vi "Get RelativePath.vi"(8 "error in (no error)":errorcluster caption="错误输入（无错误）", 11 "PanelRootNode 输入":refnum<class "PanelRootNode.lvclass"> caption="DNL_LabVIEW Object in") -> (0 "error out":errorcluster caption="错误输出", 2 "RelativePath":string, 3 "PanelRootNode 输出":refnum<class "PanelRootNode.lvclass"> caption="DNL_LabVIEW Object out")   [LabVIEW 2016, in "PanelRootNode.lvclass"]
uses:
  PanelRootNode.lvclass
  C:/Users/CL/Desktop/ZcDAQprj0811/ZcDAQprj/Modules/DAQ-Display/PanelSplitToolkit/PanelDataNode/PanelDataNode.lvclass
  PanelDataNode/PanelDataNode.lvclass/PanelDataNode.ctl
  PanelDataNode/PanelDataNode.lvclass
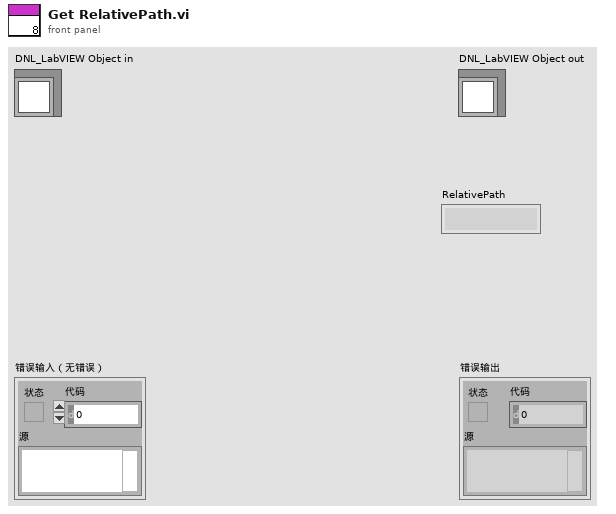
[diagram p1: front panel]
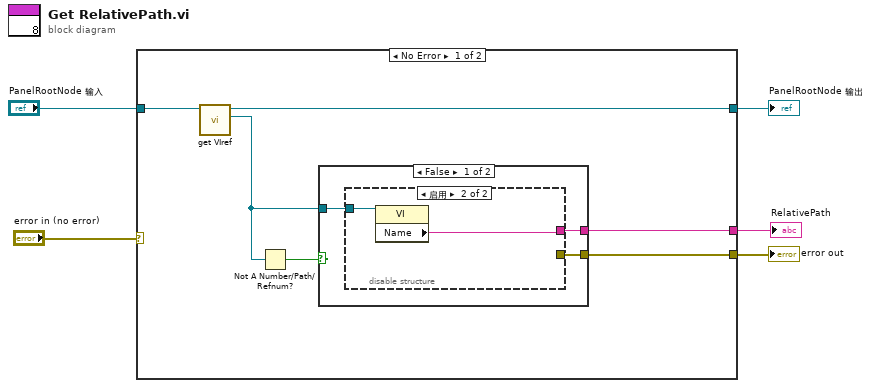
[diagram p0: block diagram]
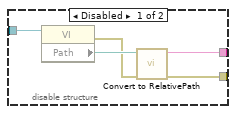
[diagram p2: hidden frame]
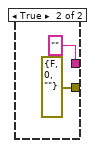
[diagram p3: hidden frame]
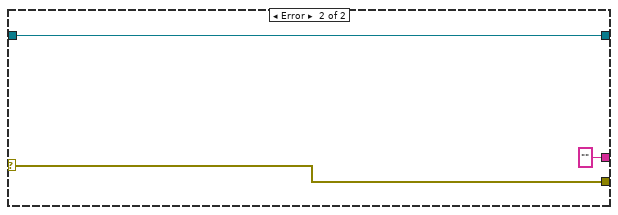
[diagram p4: hidden frame]
diagram:
  n1 = case shown="No Error" "error in (no error)" {
    selector: "error in (no error)" -> [_ w26]
    tunnel: [w6 w26] -> w4
    tunnel: [w10 w25] -> w2
    tunnel: "PanelRootNode 输入" -> [w11 w25]
    tunnel: [w7 "" ("RelativePath")] -> w1
    frame No Error {
      n2 = call "get VIref.vi"("PanelDataNode输入"=w11) -> ("VI*"=w8:refnum<vi>, "PanelDataNode输出"=w10:refnum<class "PanelRootNode.lvclass">)  [unwired: 8 in, 1 out]
      n3 = Not A Number/Path/Refnum?(number/path/refnum=w8) -> (NaN/Path/Refnum?=w9:bool)
      n4 = case shown="False" w9 {
        tunnel: w8 -> [w14 _]
        tunnel: [w13 "" ("RelativePath")] -> w7
        tunnel: [w12 errorcluster {"status"=FALSE, "code"=0, "source"=""} ("error out")] -> w6
        frame False {
          n5 = disable-structure shown="启用" {
            disable-tunnel: w14 -> [w19 w21]
            disable-tunnel: [w17 w20] -> w13
            disable-tunnel: [w16 _] -> w12
            frame Disabled {
              n6 = property class="VI"(reference=w19) -> (error out=w15:errorcluster, "Path"=w18:path)  [unwired: 1 in, 1 out]
              n7 = call "Convert to RelativePath.vi"("error in (no error)"=w15, "VI Path"=w18) -> ("error out"=w16:errorcluster, "RelativePath"=w17:string)  [unwired: 8 in]
            }
            frame Enabled {
              n8 = property class="VI"(reference=w21) -> ("Name"=w20:string)  [unwired: 1 in, 2 out]
            }
          }
        }
        frame True {
        }
      }
    }
    frame Error {
    }
  }
  "error out" <- w4
  "PanelRootNode 输出" <- w2
  "RelativePath" <- w1
